vi "Control HV PowerSupply.vi"(8 "error in":errorcluster, 9 "Socket Index":i16, 11 "PPS Config In":T1={"VISA Resource"="", "Voltage Level (0.0 V)"=0.0, "CURRent Limit (0.0 A)"=0.0, "OVP LEVEL (0V)"=0.0, "Enable OVP (T: Enable)"=TRUE, "OCP LEVEL (0A)"=0.0, "Enable OCP (T: Enable)"=TRUE, "Value Out"="", "Value In"="", "Actual Voltage Level (V)"=0.0, "Actual Current Limit (A)"=0.0, "Select Instrument"="", "Enable Output"=FALSE, "PPS Operation"=enum."Close", "Type"=0} {"Type" items=["Voltage", "Current"]; "Actual Current Limit (A)" format="%.2f"; "Actual Voltage Level (V)" format="%.2f"; "OCP LEVEL (0A)" format="%.2f"; "OVP LEVEL (0V)" format="%.2f"; "Voltage Level (0.0 V)" format="%.2f"}) -> (0 "error out":errorcluster, 2 "Report Text":string, 3 "PPS Config Out":T1={"VISA Resource"="", "Voltage Level (0.0 V)"=0.0, "CURRent Limit (0.0 A)"=0.0, "OVP LEVEL (0V)"=0.0, "Enable OVP (T: Enable)"=TRUE, "OCP LEVEL (0A)"=0.0, "Enable OCP (T: Enable)"=TRUE, "Value Out"="", "Value In"="", "Actual Voltage Level (V)"=0.0, "Actual Current Limit (A)"=0.0, "Select Instrument"="", "Enable Output"=FALSE, "PPS Operation"=enum."Close", "Type"=0} {"Type" items=["Voltage", "Current"]; "Actual Current Limit (A)" format="%.2f"; "Actual Voltage Level (V)" format="%.2f"; "OCP LEVEL (0A)" format="%.2f"; "OVP LEVEL (0V)" format="%.2f"; "Voltage Level (0.0 V)" format="%.2f"})   [LabVIEW 2023, in "HardwareAbstractionLayer_LVOOP.lvlib" / "Wait Monitor.lvclass"]
uses:
  Wait Monitor.lvclass
  PowerSupply/Teststand/Control/PPS StepType Control.ctl
  PowerSupply/IT-M6018C/IT-M6018C.lvclass
  PowerSupply/Control/PPS Configure Data.ctl
  PowerSupply/PowerSupply.lvclass
  Database/Database.lvclass
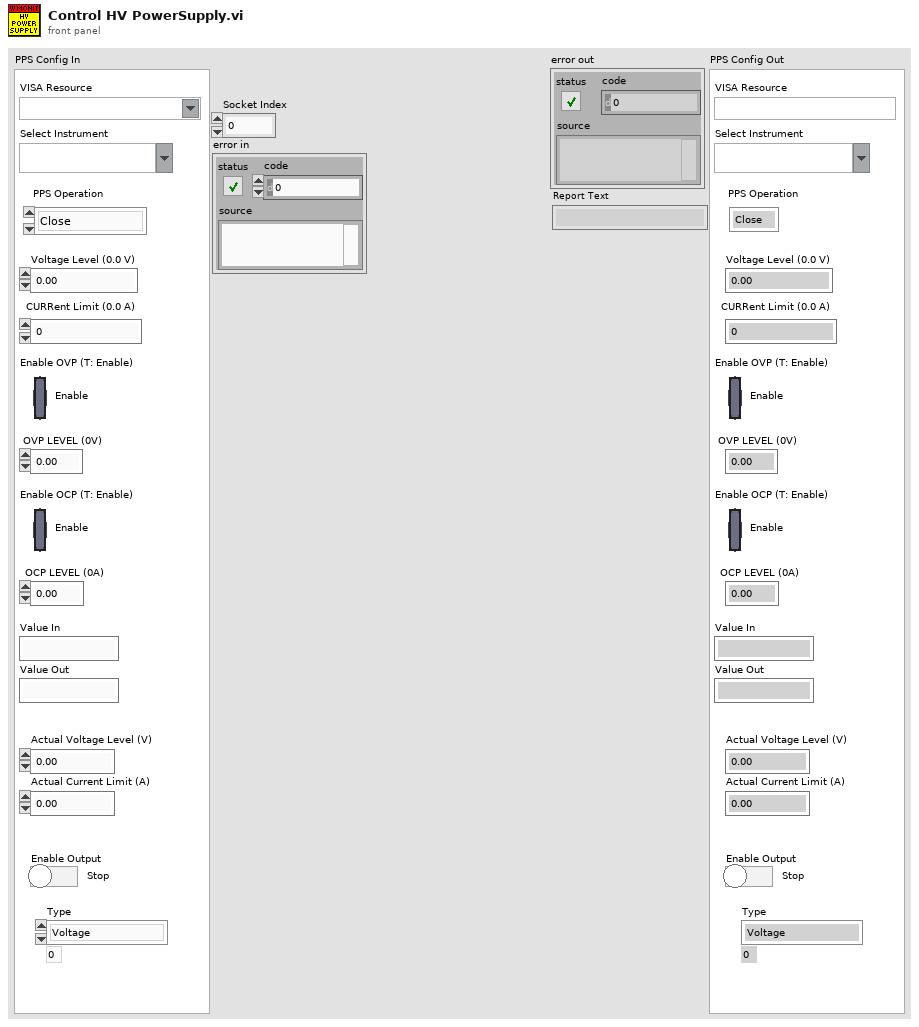
[diagram p1: front panel]
types:
  T1 = typedef "HardwareAbstractionLayer_LVOOP.lvlib/PowerSupply.lvclass/PPS StepType Control.ctl" = cluster{"VISA Resource":refnum<visa-resource-name>, "Voltage Level (0.0 V)":dbl, "CURRent Limit (0.0 A)":dbl, "OVP LEVEL (0V)":dbl, "Enable OVP (T: Enable)":bool, "OCP LEVEL (0A)":dbl, "Enable OCP (T: Enable)":bool, "Value Out":string, "Value In":string, "Actual Voltage Level (V)":dbl, "Actual Current Limit (A)":dbl, "Select Instrument":string, "Enable Output":bool, "PPS Operation":enum32{"Init", "Self Test", "Configure", "Measure", "Close"}, "Type":u16}
  T2 = typedef "HardwareAbstractionLayer_LVOOP.lvlib/PowerSupply.lvclass/PPS Configure Data.ctl" = cluster{"Voltage Level (0.0 V)":dbl, "CURRent Limit (0.0 A)":dbl, "OVP LEVEL (0V)":dbl, "OCP LEVEL (0A)":dbl, "Enable OVP (T: Enable)":bool, "Enable OCP (T: Enable)":bool, "Enable Output ":bool, "Delays OCP":dbl, "Delays OVP":dbl, "Mode(0:Voltage)":u16, "CURRent Level (0.0 A)":dbl, "Voltage Limit (0.0 V)":dbl}
  T3 = enum32{"Init", "Self Test", "Configure", "Measure", "Close"}
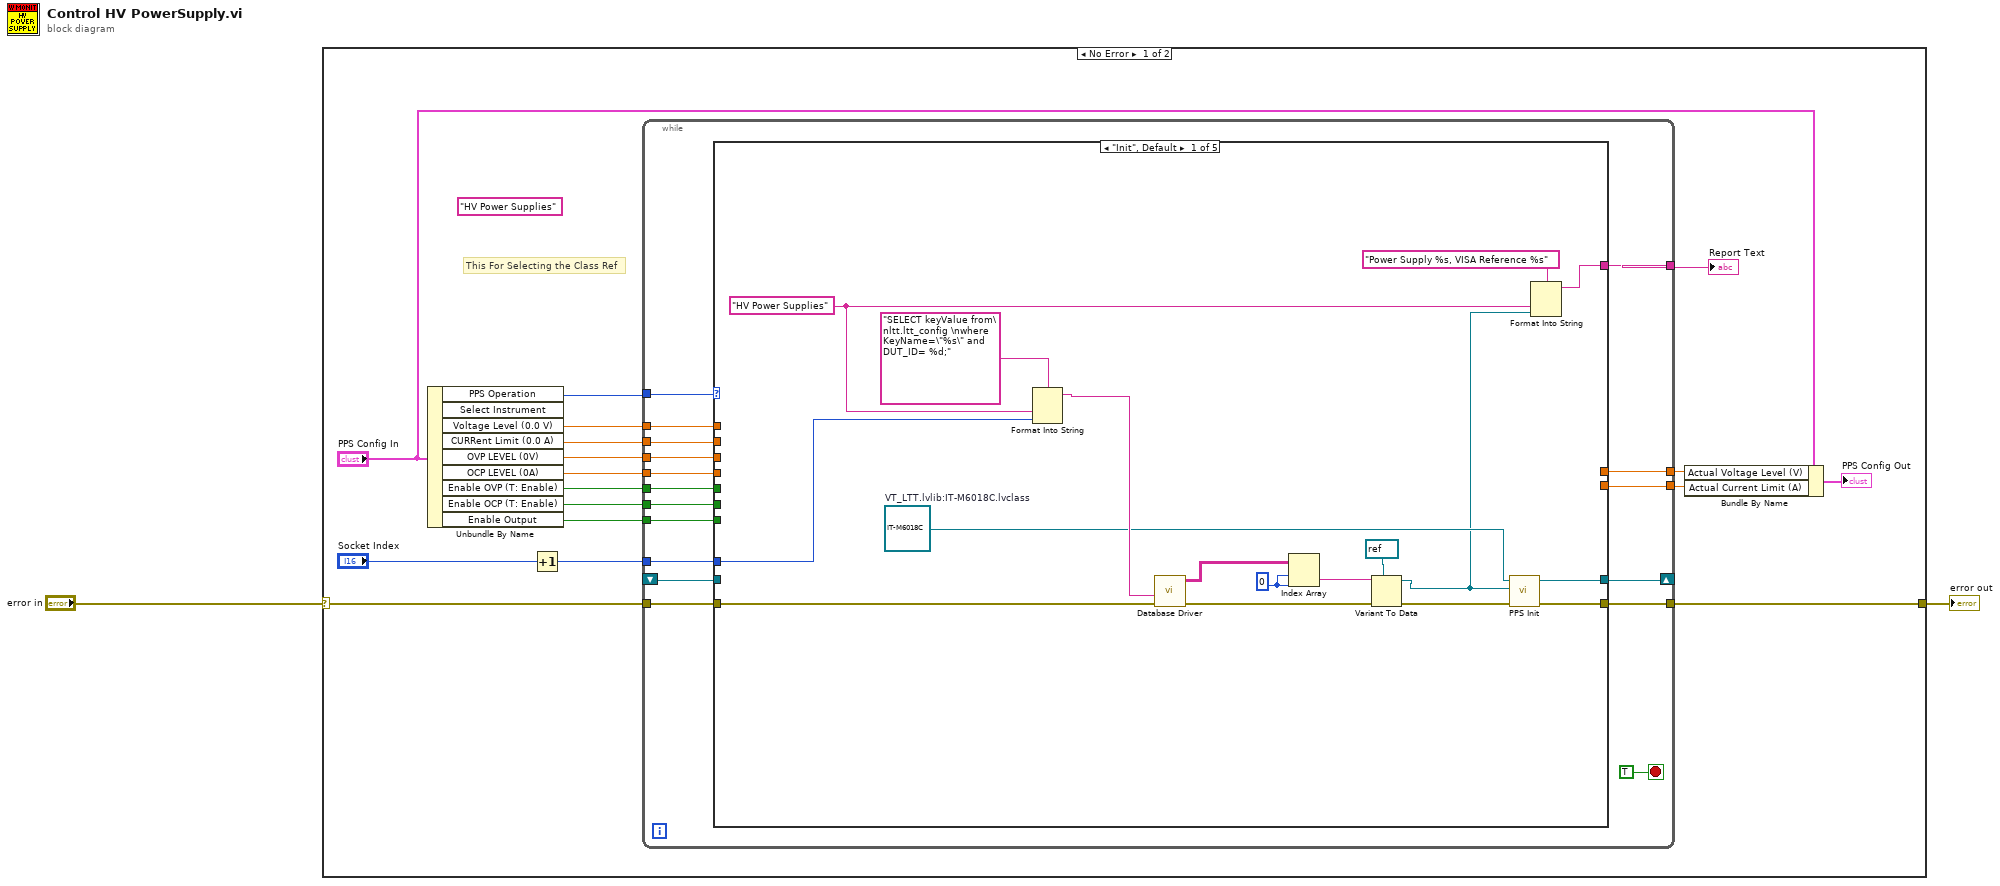
[diagram p0: block diagram]
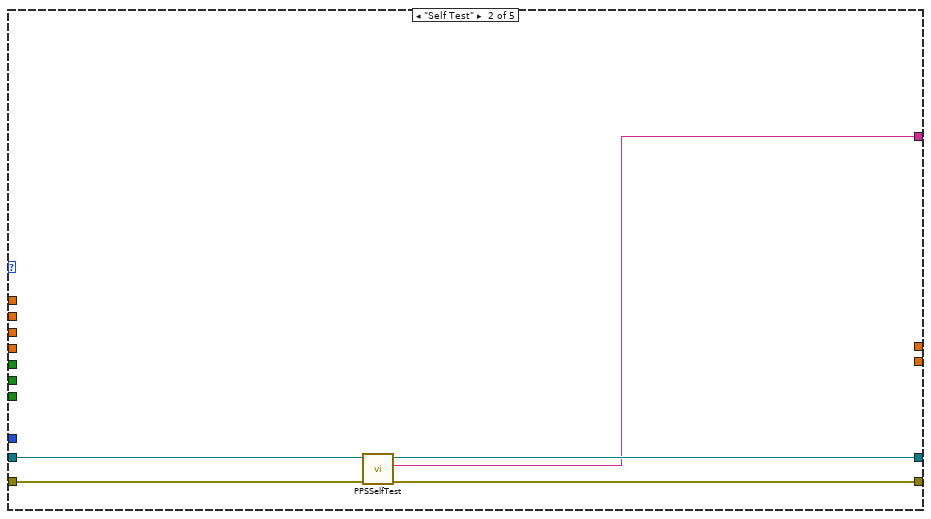
[diagram p2: hidden frame]
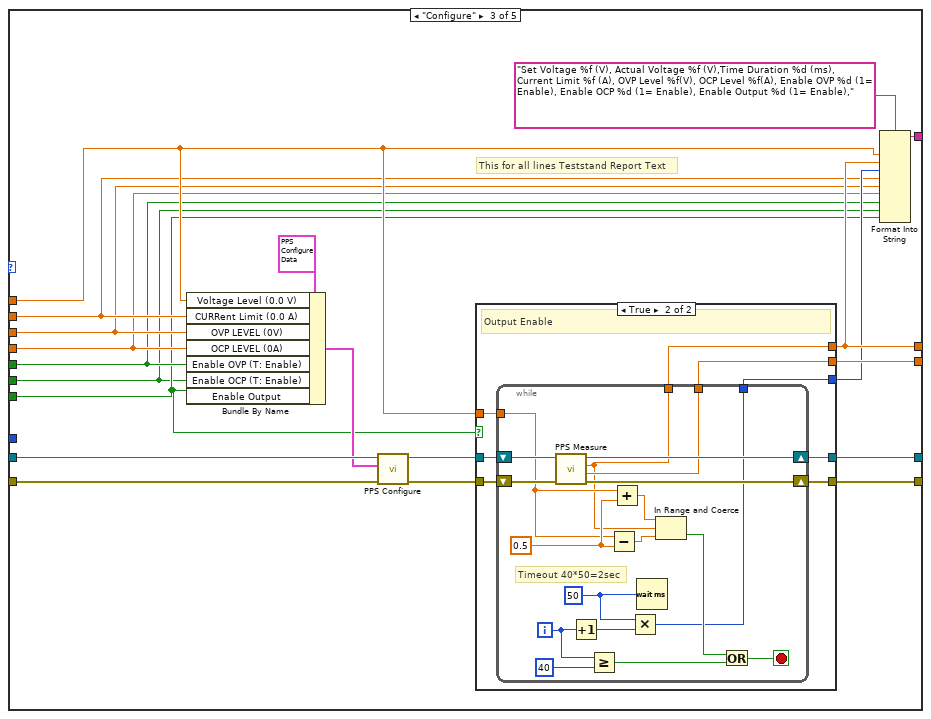
[diagram p3: hidden frame]
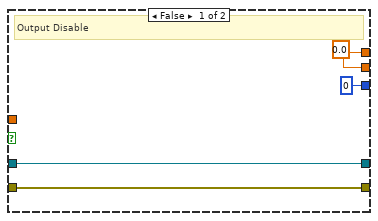
[diagram p4: hidden frame]
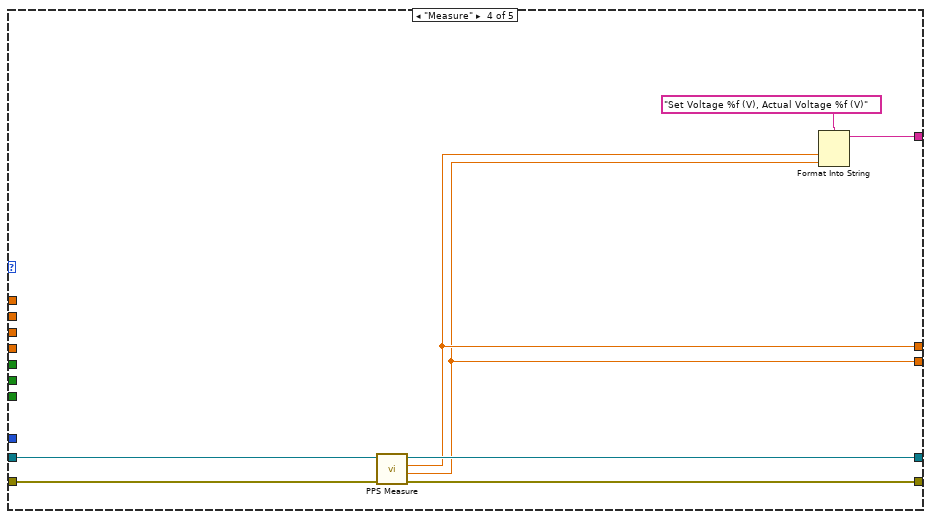
[diagram p5: hidden frame]
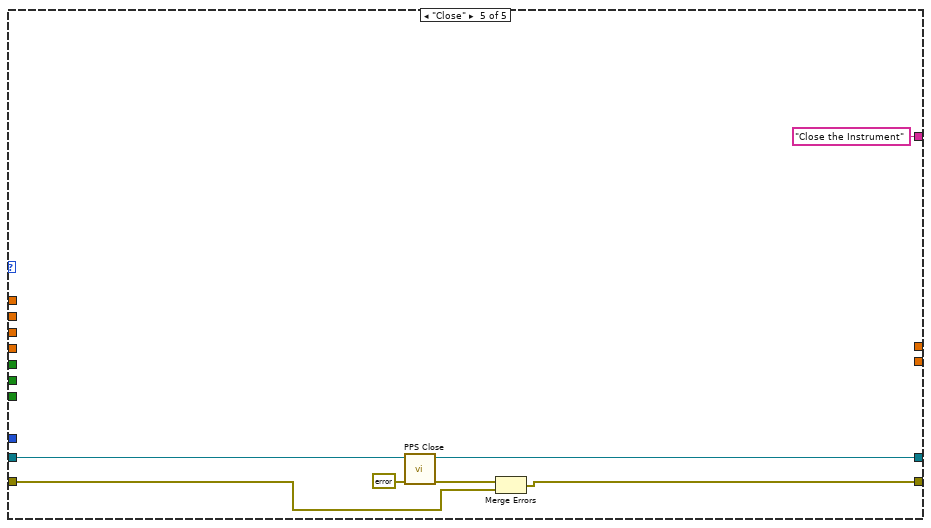
[diagram p6: hidden frame]
diagram:
  n1 = case shown="No Error" "error in" {
    selector: "error in" -> [w18 w124]
    tunnel: [w17 w124] -> w1
    frame No Error {
      (unwired) "HV Power Supplies" ("Select Instrument")
      # "This For Selecting the Class Ref"
      n2 = Unbundle By Name("PPS Config In") -> ("PPS Operation"=w19:T3, "Voltage Level (0.0 V)"=w16:dbl, "CURRent Limit (0.0 A)"=w15:dbl, "OVP LEVEL (0V)"=w14:dbl, "OCP LEVEL (0A)"=w13:dbl, "Enable OVP (T: Enable)"=w12:bool, "Enable OCP (T: Enable)"=w11:bool, "Enable Output"=w10:bool)  [unwired: 1 out]
      n3 = Increment(x="Socket Index") -> (x+1=w3:i16)
      n4 = while {
        tunnel: w19 -> [w35]
        shift-right: [w32] -> _
        shift-left: _ -> [w31]
        tunnel: w16 -> [w30]
        tunnel: w15 -> [w29]
        tunnel: w14 -> [w28]
        tunnel: w13 -> [w27]
        tunnel: w12 -> [w26]
        tunnel: w11 -> [w25]
        tunnel: w10 -> [w24]
        tunnel: w3 -> [w23]
        tunnel: [w22] -> w8
        tunnel: [w21] -> w5
        tunnel: [w20] -> w4
        tunnel: w18 -> [w34]
        tunnel: [w33] -> w17
        stop <- TRUE stop-if-true
        n5 = case shown="\"Init\", Default" w35 {
          tunnel: w34 -> [w44 w57 w77 w115 w117]
          tunnel: [w53 w56 w74 w114 w118] -> w33
          tunnel: [w52 w55 w73 w113 w121] -> w32
          tunnel: w31 -> [_ w58 w78 w116 w122]
          tunnel: w30 -> [_ _ w70 _ _]
          tunnel: w29 -> [_ _ w64 _ _]
          tunnel: w28 -> [_ _ w63 _ _]
          tunnel: w27 -> [_ _ w62 _ _]
          tunnel: w26 -> [_ _ w61 _ _]
          tunnel: w25 -> [_ _ w59 _ _]
          tunnel: w24 -> [_ _ w60 _ _]
          tunnel: w23 -> [w51 _ _ _ _]
          tunnel: [w41 w54 w69 w111 "Close the Instrument" ("Self-Test Result Message")] -> w22
          tunnel: [_ _ w68 w110 _] -> w21
          tunnel: [_ _ w67 w109 _] -> w20
          frame "Init", Default {
            w37 = "HV Power Supplies" ("input 1")
            w42 = refnum<class "IT-M6018C.lvclass"> refnum  # VT_LTT.lvlib:IT-M6018C.lvclass
            w50 = 0 ("index (row)")
            n6 = Format Into String(format string="SELECT keyValue from\nltt.ltt_config \nwhere KeyName=\"%s\" and DUT_ID= %d;", w37, w51) -> (resulting string=w46:string)  [unwired: 2 in, 1 out]
            n7 = call "Database Driver.vi"("error in"=w44, "SQL query"=w46) -> ("error out"=w43:errorcluster, "data"=w45:string[][])  [unwired: 6 in, 2 out]
            n8 = Index Array(array=w45, index (row)=w50, index (col)=w50) -> (element=w47:string)
            n9 = Variant To Data(error in=w43, type=refnum<visa-resource-name> refnum ("VISA resource name"), Variant=w47) -> (data=w39:refnum<visa-resource-name>, error out=w49:errorcluster)
            n10 = call-dynamic "PPS Init.vi"("error in (no error)"=w49, "VISA resource name"=w39, "IT-M6018C in"=w42) -> ("error out"=w53:errorcluster, "IT-M6018C out"=w52:refnum<class "IT-M6018C.lvclass">)  [unwired: 7 in]
            n11 = Format Into String(format string="Power Supply %s, VISA Reference %s", w37, w39) -> (resulting string=w41:string)  [unwired: 2 in, 1 out]
          }
          frame "Self Test" {
            n12 = call-dynamic "PPSSelfTest.vi"("error in (no error)"=w57, "PowerSupply in"=w58) -> ("error out"=w56:errorcluster, "Self-Test Result Message"=w54:string, "PowerSupply out"=w55:refnum<class "PowerSupply.lvclass">)  [unwired: 7 in]
          }
          frame "Configure" {
            # "This for all lines Teststand Report Text"
            n13 = Bundle By Name(cluster=T2 {"Voltage Level (0.0 V)"=0.0, "CURRent Limit (0.0 A)"=0.0, "OVP LEVEL (0V)"=0.0, "OCP LEVEL (0A)"=0.0, "Enable OVP (T: Enable)"=TRUE, "Enable OCP (T: Enable)"=TRUE, "Enable Output "=TRUE, "Delays OCP"=0.0, "Delays OVP"=0.0, "Mode(0:Voltage)"=0, "CURRent Level (0.0 A)"=0.0, "Voltage Limit (0.0 V)"=0.0} ("Configure"), "Voltage Level (0.0 V)"=w70, "CURRent Limit (0.0 A)"=w64, "OVP LEVEL (0V)"=w63, "OCP LEVEL (0A)"=w62, "Enable OVP (T: Enable)"=w61, "Enable OCP (T: Enable)"=w59, "Enable Output"=w60) -> (w75:T2)
            n14 = call-dynamic "PPS Configure.vi"("error in (no error)"=w77, "Configure"=w75, "PowerSupply in"=w78) -> ("error out"=w66:errorcluster, "PowerSupply out"=w72:refnum<class "PowerSupply.lvclass">)  [unwired: 7 in]
            n15 = case shown="True" w60 {
              tunnel: w66 -> [w81 w90]
              tunnel: [w81 w89] -> w74
              tunnel: [w82 w88] -> w73
              tunnel: w72 -> [w82 w87]
              tunnel: w70 -> [_ w84]
              tunnel: [w80 w86] -> w68
              tunnel: [w80 w85] -> w67
              tunnel: [u32 0 w83] -> w65
              frame False {
                w80 = 0.0 ("Actual Voltage Level (V)")
                # "Output Disable"
              }
              frame True {
                # "Output Enable"
                n16 = while {
                  tunnel: [w96] -> w86
                  tunnel: [w104] -> w85
                  shift-right: [w107] -> w89
                  shift-left: w90 -> [w108]
                  shift-right: [w106] -> w88
                  shift-left: w87 -> [w105]
                  tunnel: w84 -> [w97]
                  tunnel: [w94] -> w83
                  i -> [w93]
                  stop <- w101 stop-if-true
                  w99 = 0.5
                  w95 = u32 50 ("milliseconds to wait")
                  # "Timeout 40*50=2sec"
                  n17 = call-dynamic "PPS Measure.vi"("error in (no error)"=w108, "PowerSupply in"=w105) -> ("error out"=w107:errorcluster, "Actual Current Limit (A)"=w104:dbl, "Actual Voltage Level (V)"=w96:dbl, "PowerSupply out"=w106:refnum<class "PowerSupply.lvclass">)  [unwired: 6 in]
                  n18 = Increment(x=w93) -> (x+1=w91:i32)
                  n19 = Greater Or Equal?(x=w93, y=40) -> (x >= y?=w103:bool)
                  n20 = Subtract(x=w97, y=w99) -> (x-y=w98:dbl)
                  n21 = Add(x=w97, y=w99) -> (x+y=w100:dbl)
                  n22 = Multiply(x=w95, y=w91) -> (x*y=w94:u32)
                  n23 = Wait (ms)(milliseconds to wait=w95) -> ()  [unwired: 1 out]
                  n24 = In Range and Coerce(upper limit=w100, x=w96, lower limit=w98) -> (In Range?=w102:bool)  [unwired: 1 out]
                  n25 = Or(x=w102, y=w103) -> (x .or. y?=w101:bool)
                }
              }
            }
            n26 = Format Into String(format string="Set Voltage %f (V), Actual Voltage %f (V),Time Duration %d (ms), Current Limit %f (A), OVP Level %f(V), OCP Level %f(A), Enable OVP %d (1= Enable), Enable OCP %d (1= Enable), Enable Output %d (1= Enable),", w70, w68, w65, w64, w63, w62, w61, w59, w60) -> (resulting string=w69:string)  [unwired: 2 in, 1 out]
          }
          frame "Measure" {
            n27 = call-dynamic "PPS Measure.vi"("error in (no error)"=w115, "PowerSupply in"=w116) -> ("error out"=w114:errorcluster, "Actual Current Limit (A)"=w109:dbl, "Actual Voltage Level (V)"=w110:dbl, "PowerSupply out"=w113:refnum<class "PowerSupply.lvclass">)  [unwired: 6 in]
            n28 = Format Into String(format string="Set Voltage %f (V), Actual Voltage %f (V)", w110, w109) -> (resulting string=w111:string)  [unwired: 2 in, 1 out]
          }
          frame "Close" {
            n29 = call-dynamic "PPS Close.vi"("error in (no error)"=errorcluster {"status"=FALSE, "code"=0, "source"=""}, "PowerSupply in"=w122) -> ("error out"=w123:errorcluster, "PowerSupply out"=w121:refnum<class "PowerSupply.lvclass">)  [unwired: 8 in]
            n30 = Merge Errors(w123, w117) -> (w118:errorcluster)
          }
        }
      }
      "Report Text" <- w8
      n31 = Bundle By Name(cluster="PPS Config In", "Actual Voltage Level (V)"=w5, "Actual Current Limit (A)"=w4) -> (→"PPS Config Out":T1)
    }
    frame Error {
    }
  }
  "error out" <- w1
